vi "Problem1.5.vi"() -> ()   [LabVIEW 2019]
panel:
  in  "Reset":bool
  in  "Set":bool
  out "Output":bool
  out "Output Negation":bool
  # "SR Flip Flop"
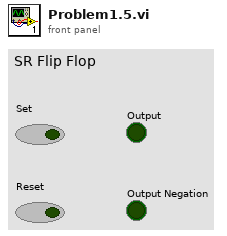
[diagram p1: front panel]
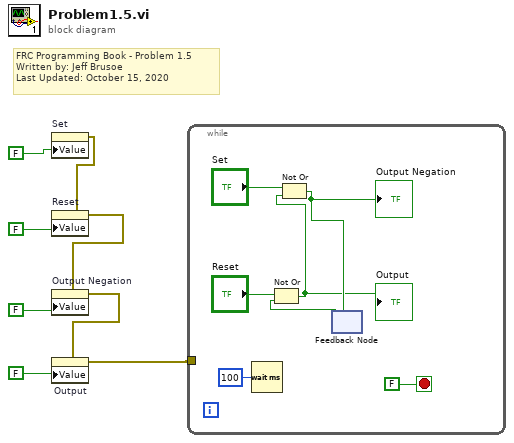
[diagram p0: block diagram]
diagram:
  # "FRC Programming Book - Problem 1.5\nWritten by: Jeff Brusoe\nLast Updated: October 15, 2020"
  n1 = property on="Set" class="Bool (strict)"("Value"=FALSE ("Set")) -> (error out=w4:errorcluster)  [unwired: 2 in, 1 out]
  n2 = property on="Reset" class="Bool (strict)"(error in=w4, "Value"=FALSE ("Reset")) -> (error out=w3:errorcluster)  [unwired: 1 in, 1 out]
  n3 = property on="Output Negation" class="Bool (strict)"(error in=w3, "Value"=FALSE ("Output")) -> (error out=w2:errorcluster)  [unwired: 1 in, 1 out]
  n4 = property on="Output" class="Bool (strict)"(error in=w2, "Value"=FALSE ("Output Negation")) -> (error out=w1:errorcluster)  [unwired: 1 in, 1 out]
  n5 = while {
    tunnel: w1 -> [_]
    stop <- FALSE stop-if-true
    n6 = Wait (ms)(milliseconds to wait=u32 100) -> ()  [unwired: 1 out]
    n7 = feedback #1() -> (w11:bool)  [unwired: 1 in]
    n8 = Not Or(1:w11, 2:"Reset") -> (0:w9:bool)
    "Output" <- w9
    n9 = Not Or(1:w9, 2:"Set") -> (0:w10:bool)
    "Output Negation" <- w10
    n10 = feedback-in #1(w10) -> ()
  }
